vi "CRYRename All.vi"() -> (1 "Rename?":bool=TRUE, 2 "Renamed Rows":i32[](array[numeric]))   [LabVIEW 2013]
uses:
  Global/CRYCurve Library Global.vi
panel:
  # "Rename All Data(Curves, Values, Results, Waveforms)"
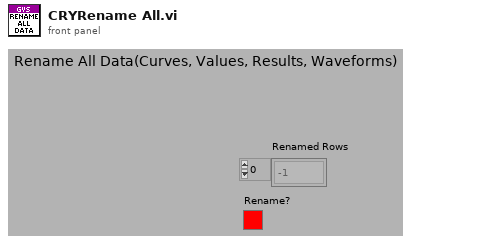
[diagram p1: front panel]
types:
  T1 = typedef "CRYData Cluster.ctl" = cluster{"Name":string, "Curve":cluster{"x":dbl, "y":dbl, "z":dbl}[], "X data":u16, "Y data":u16, "Z data":u16, "X axis":u16, "Y axis":u16, "Z axis":u16, "X unit":string, "Y unit":string, "Z unit":string, "X dB ref":dbl, "Y dB ref":dbl, "Z dB ref":dbl, "single val":bool, "protected":bool, "display X":bool, "display Y":bool, "display Z":bool, "Test Info":string, "Step No.":i32, "Plot Settings":cluster{"Color":u32, "Interpolation":u8, "Point Style":u8, "Line Style":u8, "Point Color":u32, "Line Width":u8, "Bar Plot Style":u8, "Fill To":i16}, "AutoProtect":bool}
  T2 = typedef "CRYWaveform Cluster.ctl" = cluster{"Waveform":cluster{"X0":dbl, "dX":dbl, "Y":sgl[]}, "X data":u16, "Y data":u16, "Y axis":u16, "X unit":string, "Y unit":string, "Y dB ref":dbl, "display Y":bool, "display X":bool, "Overload?":bool, "Test Info":string, "Step No.":i32, "Name":string, "protected":bool, "Sqc history":string[], "Signal Channel ID":i32, "Plot Settings":cluster{"Color":u32, "Interpolation":u8, "Point Style":u8, "Line Style":u8, "Point Color":u32, "Line Width":u8, "Bar Plot Style":u8, "Fill To":i16}, "AutoProtect":bool}
  T3 = typedef "CRYResult Cluster.ctl" = cluster{"Name":string, "Margin":dbl, "unit":string, "Verdict":bool, "Limit":string, "Max/Min":string, "protected":bool, "Step No.":i32, "Test Info":string, "AutoProtect":bool}
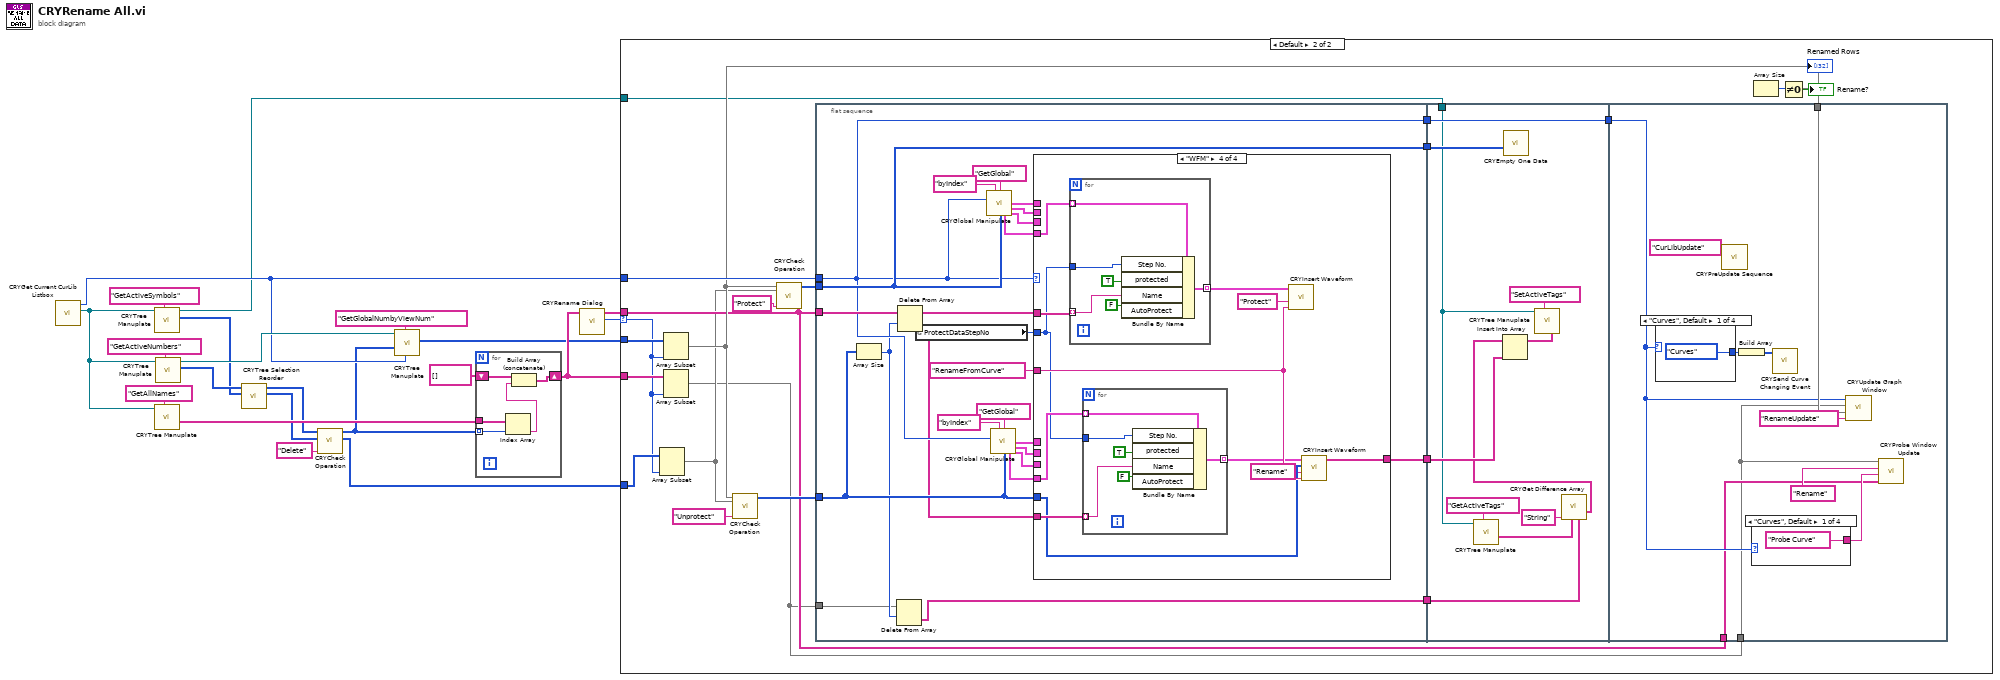
[diagram p0: block diagram]
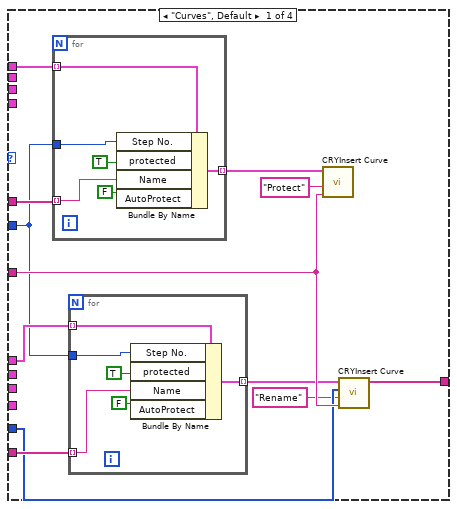
[diagram p3: hidden frame]
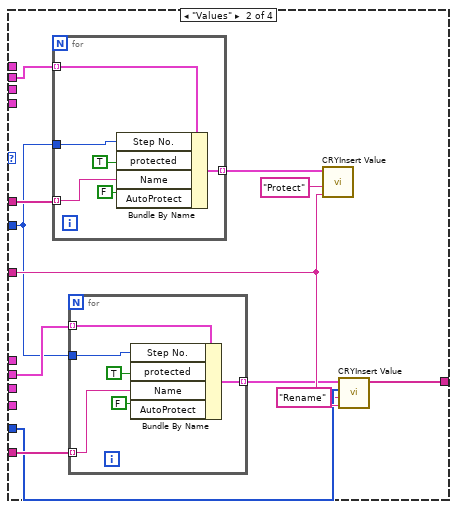
[diagram p4: hidden frame]
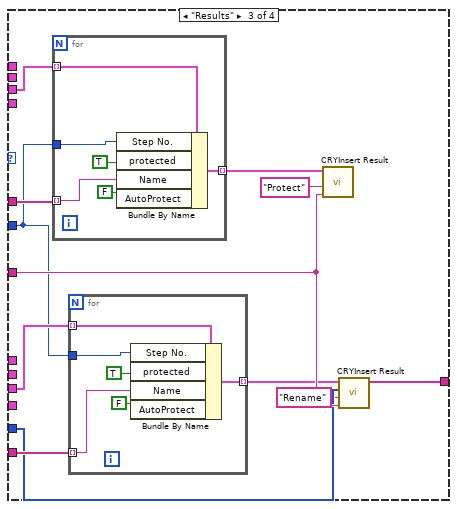
[diagram p5: hidden frame]
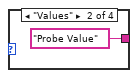
[diagram p6: hidden frame]
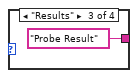
[diagram p7: hidden frame]
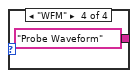
[diagram p8: hidden frame]
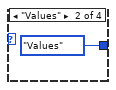
[diagram p9: hidden frame]
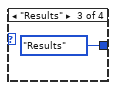
[diagram p10: hidden frame]
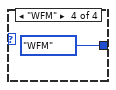
[diagram p11: hidden frame]
diagram:
  n1 = call "CRYGet Current CurLib Listbox.vi"() -> ("CurLib Tree"=w12:refnum<vi>, "Type"=w8:enum16{"Curves", "Values", "Results", "WFM"})  [unwired: 9 in, 1 out]
  n2 = call "CRYTree Manuplate.vi"("sAction"="GetActiveSymbols", "Tree in"=w12) -> ("nData Out"=w2:i32[], "Tree Out"=w5:refnum<vi>)  [unwired: 6 in, 2 out]
  n3 = call "CRYTree Manuplate.vi"("sAction"="GetAllNames", "Tree in"=w12) -> ("sData Out"=w13:string[])  [unwired: 6 in, 3 out]
  n4 = call "CRYTree Manuplate.vi"("sAction"="GetActiveNumbers", "Tree in"=w12) -> ("nData Out"=w4:i32[], "Tree Out"=w10:refnum<vi>)  [unwired: 6 in, 2 out]
  n5 = call "CRYTree Selection Reorder.vi"("Symbol In"=w2, "Number In"=w4) -> ("Symbol Out"=w1:i32[], "Number Out"=w3:i32[])  [unwired: 8 in]
  n6 = call "CRYCheck Operation.vi"("Operation"="Delete", "Item Symbols In"=w1, "Index Array In"=w3) -> ("Item Symbols Out"=w6:i32[], "Array Out"=w7:i32[])  [unwired: 1 in, 6 out]
  n7 = call "CRYTree Manuplate.vi"("Type"=w8, "sAction"="GetGlobalNumbyViewNum", "nData"=w7, "Tree in"=w10) -> ("nData Out"=w9:i32[])  [unwired: 4 in, 3 out]
  n8 = for {
    tunnel: w13 -> [w25]
    shift-right: [w23] -> w18
    shift-left: string[] [] ("subarray") -> [w24]
    tunnel: w7 -> [w26] mode=indexing
    n9 = Index Array(array=w25, index=w26) -> (element=w22:string)
    n10 = Build Array (concatenate)(w24, w22) -> (w23:string[])
  }
  n11 = call "CRYRename Dialog.vi"("Name In"=w18) -> ("Index"=w17:i32, "New Name"=w20:string[])  [unwired: 3 in, 5 out]
  n12 = case shown="Default" w17 {
    selector: w17 -> [_ w32]
    tunnel: w20 -> [_ w37]
    tunnel: w9 -> [_ w41]
    tunnel: w8 -> [_ w40]
    tunnel: w18 -> [_ w39]
    tunnel: w6 -> [_ w33]
    tunnel: w5 -> [_ w29]
    frame 0 {
    }
    frame Default {
      n13 = Array Subset(array=w33, length=w32) -> (w31:i32[])  [unwired: 1 in]
      n14 = Array Subset(array=w41, length=w32) -> (w38:i32[])  [unwired: 1 in]
      "Renamed Rows" <- w38
      n15 = Array Subset(array=w39, length=w32) -> (w27:string[])  [unwired: 1 in]
      n16 = call "CRYCheck Operation.vi"("Operation"="Unprotect", "Item Symbols In"=w31, "Index Array In"=w38) -> ("Array Out"=w47:i32[])  [unwired: 6 in, 2 out]
      n17 = call "CRYCheck Operation.vi"("Operation"="Protect", "Item Symbols In"=w31, "Index Array In"=w38) -> ("Array Out"=w46:i32[])  [unwired: 6 in, 2 out]
      n18 = flat-sequence {
        tunnel: [w59] -> w36
        tunnel: w46 -> [w62]
        tunnel: w47 -> [w58]
        tunnel: w40 -> [w59]
        tunnel: w37 -> [w70]
        tunnel: [w62] -> w34
        tunnel: [w53] -> w30
        tunnel: [w49] -> w28
        tunnel: w27 -> [w50]
        tunnel: w36 -> [w178]
        tunnel: [w178] -> w35
        tunnel: w34 -> [w177]
        tunnel: w30 -> [w176]
        tunnel: w29 -> [w168]
        tunnel: w28 -> [w170]
        tunnel: w35 -> [w181]
        tunnel: w27 -> [w179]
        tunnel: w38 -> [w183]
        tunnel: w37 -> [w180]
        frame #0 {
          n19 = Array Size(array=w58) -> (size(s)=w51:i32)
          n20 = Delete From Array(array=w50, length=w51) -> (deleted portion=w49:string[])  [unwired: 1 in, 1 out]
          n21 = Delete From Array(array=w70, length=w51) -> (deleted portion=w52:string[], array with subset deleted=w69:string[])  [unwired: 1 in]
          n22 = global read "CRYCurve Library Global.vi" "ProtectDataStepNo"() -> (w48:i32)
          n23 = call "CRYGlobal Manipulate.vi"("Type"=w59, "sOption"="byIndex", "sAction"="GetGlobal", "nData"=w62) -> ("Curves Out"=w66:T1[], "Values Out"=w65:T1[], "WFM Out"=w63:T2[], "Results Out"=w64:T3[])  [unwired: 5 in, 3 out]
          n24 = call "CRYGlobal Manipulate.vi"("Type"=w59, "sOption"="byIndex", "sAction"="GetGlobal", "nData"=w58) -> ("Curves Out"=w57:T1[], "Values Out"=w56:T1[], "WFM Out"=w54:T2[], "Results Out"=w55:T3[])  [unwired: 5 in, 3 out]
          n25 = case shown="\"WFM\"" w59 {
            tunnel: w69 -> [w83 w107 w131 w155]
            tunnel: w58 -> [w75 w101 w127 w151]
            tunnel: w52 -> [w82 w106 w130 w154]
            tunnel: "RenameFromCurve" ("sOption") -> [w77 w103 w128 w152]
            tunnel: w66 -> [w81 _ _ _]
            tunnel: w65 -> [_ w100 _ _]
            tunnel: w64 -> [_ _ w126 _]
            tunnel: w63 -> [_ _ _ w150]
            tunnel: w57 -> [w80 _ _ _]
            tunnel: w56 -> [_ w99 _ _]
            tunnel: w55 -> [_ _ w124 _]
            tunnel: w54 -> [_ _ _ w149]
            tunnel: [w73 w97 w121 w145] -> w53
            tunnel: w48 -> [w72 w96 w120 w144]
            frame "Curves", Default {
              n26 = for {
                tunnel: w83 -> [w94] mode=indexing
                tunnel: w81 -> [w92] mode=indexing
                tunnel: [w91] -> w78 mode=indexing
                tunnel: w72 -> [w90]
                n27 = Bundle By Name(cluster=w92, "Step No."=w90, "protected"=TRUE, "Name"=w94, "AutoProtect"=FALSE) -> (w91:T1)
              }
              n28 = for {
                tunnel: w82 -> [w88] mode=indexing
                tunnel: w80 -> [w86] mode=indexing
                tunnel: [w85] -> w76 mode=indexing
                tunnel: w72 -> [w84]
                n29 = Bundle By Name(cluster=w86, "Step No."=w84, "protected"=TRUE, "Name"=w88, "AutoProtect"=FALSE) -> (w85:T1)
              }
              n30 = call "CRYInsert Curve.vi"("sOptionUpdate"=w77, "sOption"="Protect", "Curve"=w78) -> ()  [unwired: 1 in, 8 out]
              n31 = call "CRYInsert Curve.vi"("sOptionUpdate"=w77, "sOption"="Rename", "Index"=w75, "Curve"=w76) -> ("Inserted Name Out"=w73:string[])  [unwired: 7 out]
            }
            frame "Values" {
              n32 = for {
                tunnel: w107 -> [w118] mode=indexing
                tunnel: w100 -> [w116] mode=indexing
                tunnel: [w115] -> w104 mode=indexing
                tunnel: w96 -> [w114]
                n33 = Bundle By Name(cluster=w116, "Step No."=w114, "protected"=TRUE, "Name"=w118, "AutoProtect"=FALSE) -> (w115:T1)
              }
              n34 = for {
                tunnel: w106 -> [w112] mode=indexing
                tunnel: w99 -> [w110] mode=indexing
                tunnel: [w109] -> w102 mode=indexing
                tunnel: w96 -> [w108]
                n35 = Bundle By Name(cluster=w110, "Step No."=w108, "protected"=TRUE, "Name"=w112, "AutoProtect"=FALSE) -> (w109:T1)
              }
              n36 = call "CRYInsert Value.vi"("sOptionUpdate"=w103, "sOption"="Protect", "Value"=w104) -> ()  [unwired: 7 in, 2 out]
              n37 = call "CRYInsert Value.vi"("sOptionUpdate"=w103, "sOption"="Rename", "Index"=w101, "Value"=w102) -> ("Inserted Name Out"=w97:string[])  [unwired: 6 in, 1 out]
            }
            frame "Results" {
              n38 = for {
                tunnel: w131 -> [w142] mode=indexing
                tunnel: w126 -> [w140] mode=indexing
                tunnel: [w139] -> w125 mode=indexing
                tunnel: w120 -> [w138]
                n39 = Bundle By Name(cluster=w140, "Step No."=w138, "protected"=TRUE, "Name"=w142, "AutoProtect"=FALSE) -> (w139:T3)
              }
              n40 = for {
                tunnel: w130 -> [w136] mode=indexing
                tunnel: w124 -> [w134] mode=indexing
                tunnel: [w133] -> w123 mode=indexing
                tunnel: w120 -> [w132]
                n41 = Bundle By Name(cluster=w134, "Step No."=w132, "protected"=TRUE, "Name"=w136, "AutoProtect"=FALSE) -> (w133:T3)
              }
              n42 = call "CRYInsert Result.vi"("sOptionUpdate"=w128, "sOption"="Protect", "Result"=w125) -> ()  [unwired: 7 in, 2 out]
              n43 = call "CRYInsert Result.vi"("sOptionUpdate"=w128, "sOption"="Rename", "Index"=w127, "Result"=w123) -> ("Inserted Name Out"=w121:string[])  [unwired: 6 in, 1 out]
            }
            frame "WFM" {
              n44 = for {
                tunnel: w155 -> [w166] mode=indexing
                tunnel: w150 -> [w164] mode=indexing
                tunnel: [w163] -> w147 mode=indexing
                tunnel: w144 -> [w162]
                n45 = Bundle By Name(cluster=w164, "Step No."=w162, "protected"=TRUE, "Name"=w166, "AutoProtect"=FALSE) -> (w163:T2)
              }
              n46 = for {
                tunnel: w154 -> [w160] mode=indexing
                tunnel: w149 -> [w158] mode=indexing
                tunnel: [w157] -> w148 mode=indexing
                tunnel: w144 -> [w156]
                n47 = Bundle By Name(cluster=w158, "Step No."=w156, "protected"=TRUE, "Name"=w160, "AutoProtect"=FALSE) -> (w157:T2)
              }
              n48 = call "CRYInsert Waveform.vi"("sOptionUpdate"=w152, "sOption"="Protect", "Waveform"=w147) -> ()  [unwired: 7 in, 2 out]
              n49 = call "CRYInsert Waveform.vi"("sOptionUpdate"=w152, "sOption"="Rename", "Index"=w151, "Waveform"=w148) -> ("Inserted Name Out"=w145:string[])  [unwired: 6 in, 1 out]
            }
          }
        }
        frame #1 {
          n50 = call "CRYTree Manuplate.vi"("sAction"="GetActiveTags", "Tree in"=w168) -> ("sData Out"=w171:string[])  [unwired: 6 in, 3 out]
          n51 = call "CRYEmpty One Data.vi"("Index"=w177) -> ()  [unwired: 2 in, 9 out]
          n52 = call "CRYGet Difference Array.vi"("String2"=w170, "String1"=w171, "sOption"="String") -> ("StringDiff Out"=w169:string[])  [unwired: 7 in, 1 out]
          n53 = Insert Into Array(array=w169, new element=w176) -> (w174:string[])  [unwired: 1 in]
          n54 = call "CRYTree Manuplate.vi"("sData"=w174, "sAction"="SetActiveTags", "Tree in"=w168) -> ()  [unwired: 5 in, 4 out]
        }
        frame #2 {
          n55 = case shown="\"Curves\", Default" w181 {
            tunnel: [enum16{"Curves", "Values", "Results", "WFM"}."Curves" ("Type In") enum16{"Curves", "Values", "Results", "WFM"}."Values" ("Type In") enum16{"Curves", "Values", "Results", "WFM"}."Results" ("Type In") enum16{"Curves", "Values", "Results", "WFM"}."WFM" ("Type In")] -> w186
            frame "Curves", Default {
            }
            frame "Values" {
            }
            frame "Results" {
            }
            frame "WFM" {
            }
          }
          n56 = call "CRYPreUpdate Sequence.vi"("EventName"="CurLibUpdate") -> ()  [unwired: 15 in]
          n57 = Build Array(w186) -> (w185:enum16{"Curves", "Values", "Results", "WFM"}[])
          n58 = case shown="\"Curves\", Default" w181 {
            tunnel: ["Probe Curve" "Probe Value" "Probe Result" "Probe Waveform"] -> w182
            frame "Curves", Default {
            }
            frame "Values" {
            }
            frame "Results" {
            }
            frame "WFM" {
            }
          }
          n59 = call "CRYSend Curve Changing Event.vi"("Type"=w185) -> ()  [unwired: 11 out]
          n60 = call "CRYUpdate Graph Window.vi"("sOption"="RenameUpdate", "Index"=w183, "Del/Update Names"=w179, "Type"=w181) -> ()  [unwired: 8 out]
          n61 = call "CRYProbe Window Update.vi"("NamesforRename"=w180, "ProbeType"=w182, "sAction"="Rename", "Names"=w179) -> ()  [unwired: 8 out]
        }
      }
      n62 = Array Size(array=w38) -> (size(s)=w45:i32)
      n63 = Not Equal To 0?(x=w45) -> (x != 0?=→"Rename?":bool)
    }
  }
